vi "DoProcess.vi"(8 "error in (no error)":errorcluster, 9 "MsgQ":refnum<queue>, 10 "AbstractionActor.lvclass":refnum<class "AbstractionActor.lvclass">, 11 "AbstractionMessage in":refnum<class "AbstractionMessage.lvclass">) -> (0 "error out":errorcluster, 2 "AbstractionActor.lvclass 2":refnum<class "AbstractionActor.lvclass">, 3 "AbstractionMessage out":refnum<class "AbstractionMessage.lvclass">)   [LabVIEW 2021, in "AbstractionMessage.lvclass"]
uses:
  AbstractionMessage.lvclass
  AbstractionActor/AbstractionActor.lvclass
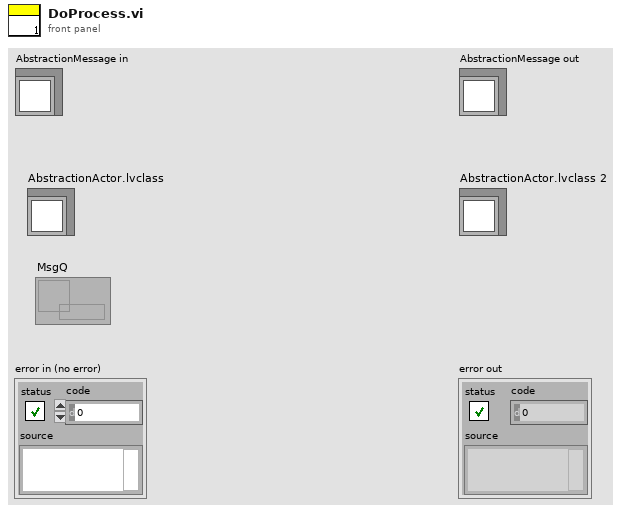
[diagram p1: front panel]
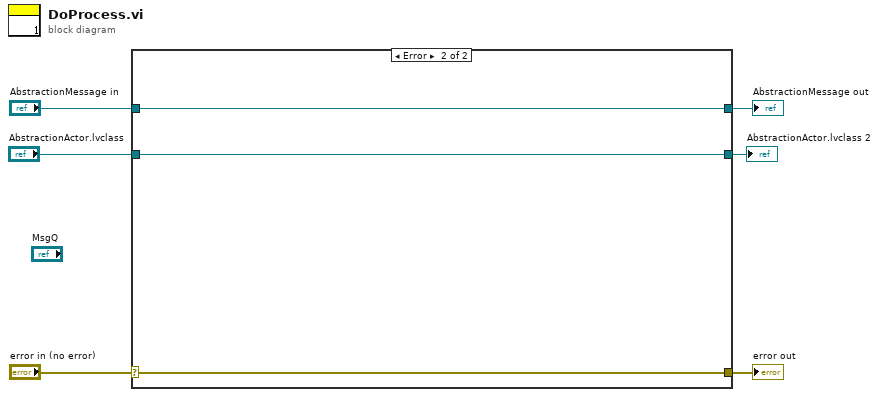
[diagram p0: block diagram]
diagram:
  n1 = case shown="Error" "error in (no error)" {
    selector: "error in (no error)" -> [w8 w12]
    tunnel: [w8 w12] -> w5
    tunnel: [w9 w11] -> w3
    tunnel: "AbstractionMessage in" -> [w9 w11]
    tunnel: [w7 w10] -> w2
    tunnel: "AbstractionActor.lvclass" -> [w7 w10]
    frame No Error {
      # "Wire the error cluster across even in the \"No Error\"\ncase so that warnings get propagated."
    }
    frame Error {
    }
  }
  "error out" <- w5
  "AbstractionMessage out" <- w3
  "AbstractionActor.lvclass 2" <- w2
